vi "rise.vi"(11 "Signal":bool) -> (3 "Count?":bool)   [LabVIEW 2017]
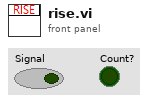
[diagram p1: front panel]
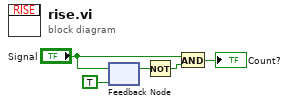
[diagram p0: block diagram]
diagram:
  n1 = feedback-in #1("Signal") -> ()
  n2 = feedback #1(TRUE ("Signal")) -> (w3:bool)
  n3 = Not(x=w3) -> (.not. x?=w4:bool)
  n4 = And(x="Signal", y=w4) -> (x .and. y?=→"Count?":bool)
